vi "Challenge 2.vi"() -> ()   [LabVIEW 2019]
panel:
  out "Brief Description of Current State":string
  in  "Limit Switch":bool
  out "Locking Pin":bool
  out "Kicker Piston":bool
  in  "Kick the Ball":bool
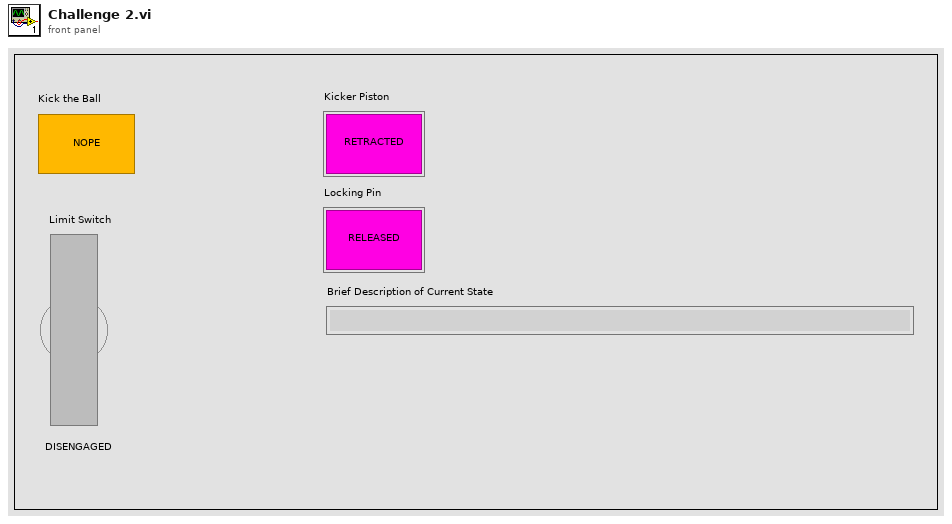
[diagram p1: front panel]
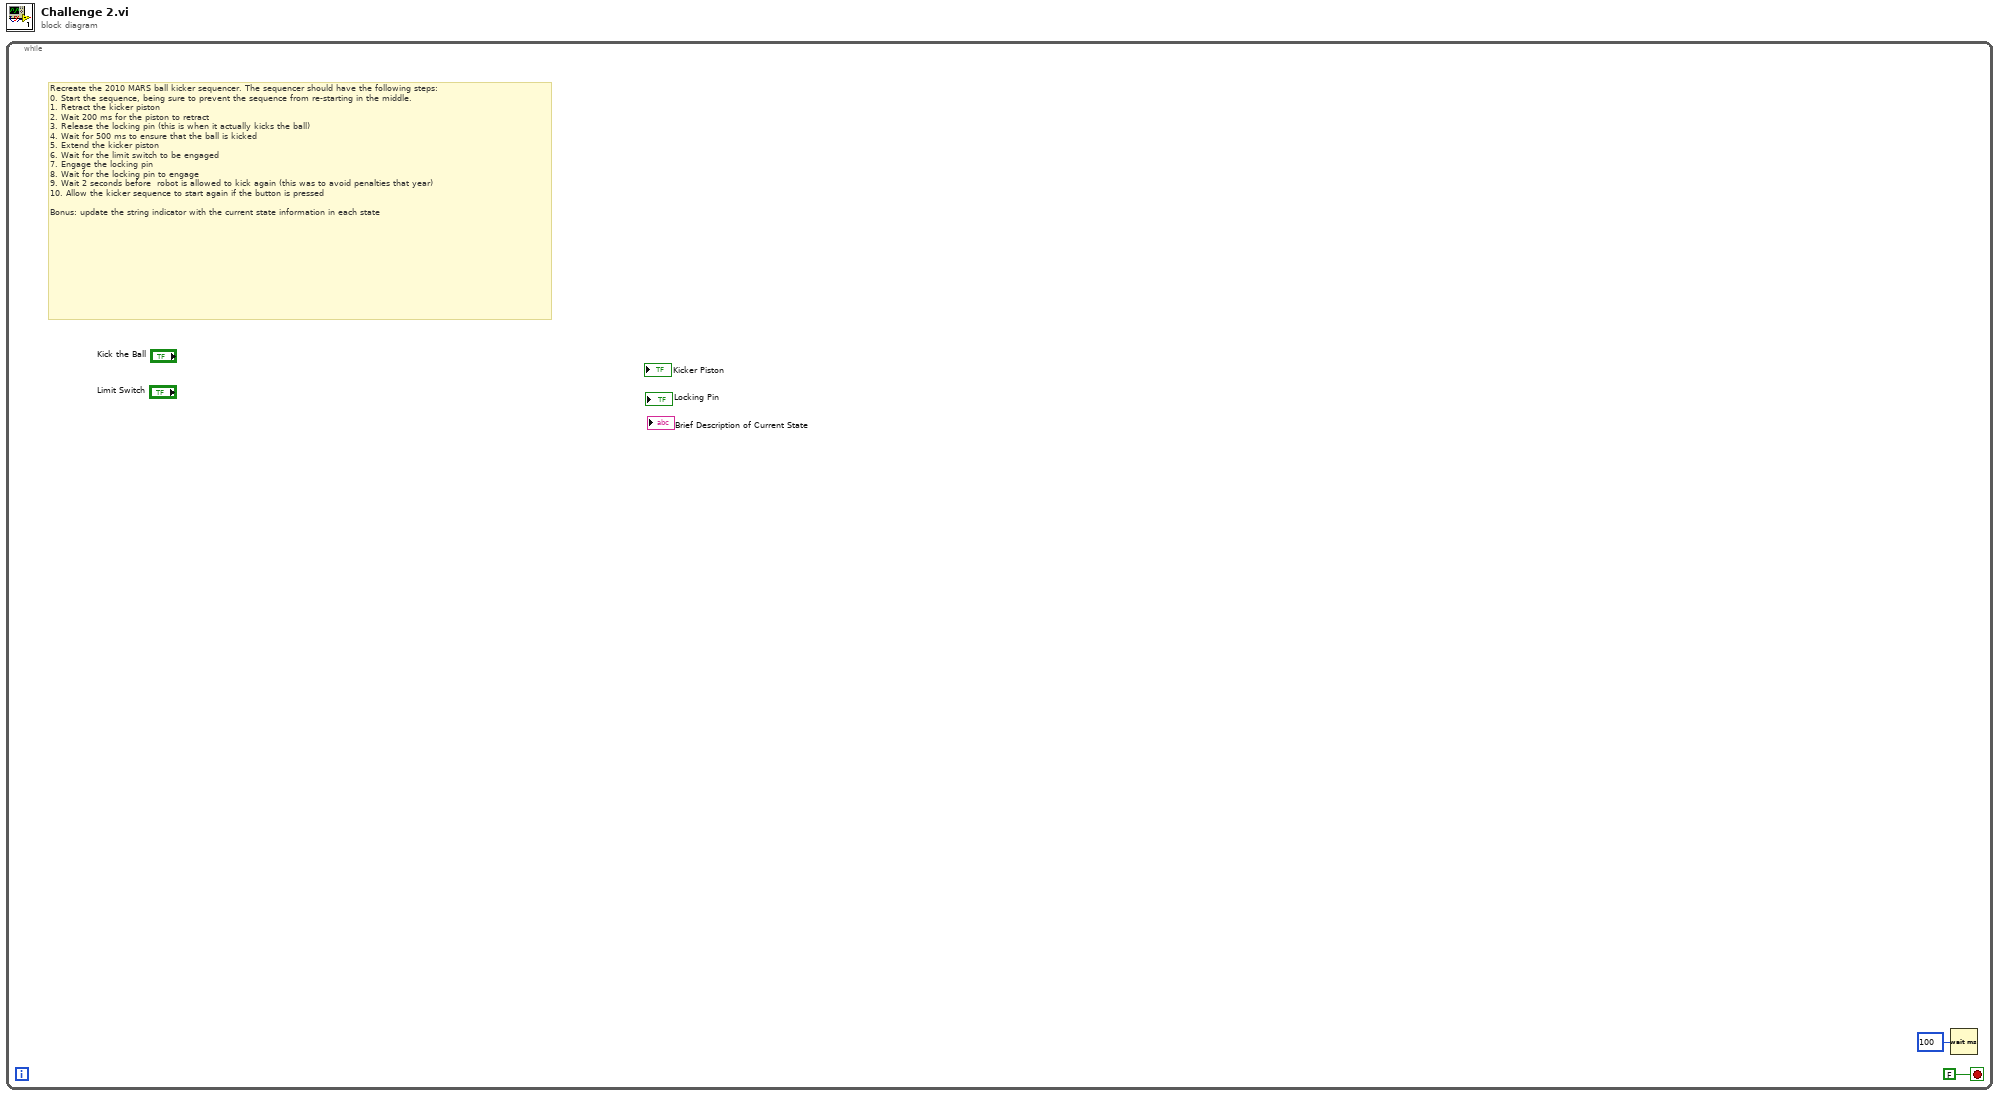
[diagram p0: block diagram]
diagram:
  n1 = while {
    stop <- FALSE stop-if-true
    # "Recreate the 2010 MARS ball kicker sequencer. The sequencer should have the following steps:\n0. Start the sequence, being sure to prevent the sequence from re-starting in the middle.\n1. Retract the kicker piston\n2. Wait 200 ms for the piston to retract\n3. Release the locking pin (this is when it actually kicks the ball)\n4. Wait for 500 ms to ensure that the ball is kicked\n5. Extend the kicker piston\n6. Wait for the limit switch to be engaged\n7. Engage the locking pin \n8. Wait for the locking pin to engage\n9. Wait 2 seconds before  robot is allowed to kick again (this was to avoid penalties that year)\n10. Allow the kicker sequence to start again if the button is pressed\n\nBonus: update the string indicator with the current state information in each state"
    n2 = Wait (ms)(milliseconds to wait=u32 100) -> ()  [unwired: 1 out]
  }
